vi "PeakFinder.vi"(9 "Trigger location":i32, 11 "Input Y values":dbl[](array[numeric])) -> (2 "peak?":bool, 3 "Input Y values":dbl[](array[numeric]))   [LabVIEW 2014]
panel:
  # "Peak Finder VI"
  # "Inputs"
  # "Outputs"
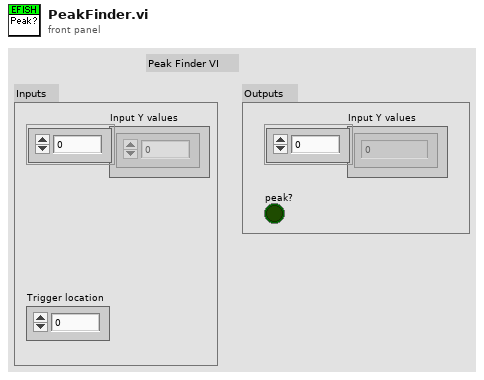
[diagram p1: front panel]
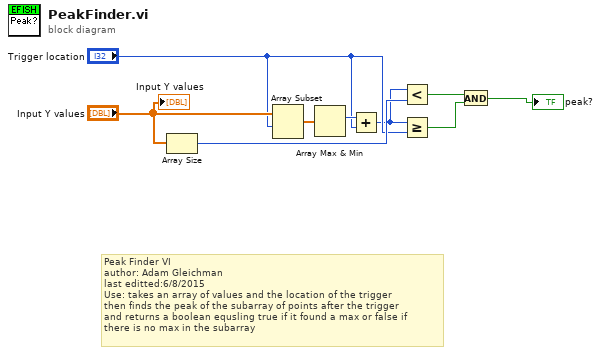
[diagram p0: block diagram]
diagram:
  # "Peak Finder VI\nauthor: Adam Gleichman\nlast editted:6/8/2015\nUse: takes an array of values and the location of the trigger\nthen finds the peak of the subarray of points after the trigger\nand returns a boolean equsling true if it found a max or false if \nthere is no max in the subarray"
  n1 = Array Size(array="Input Y values") -> (size(s)=w4:i32)
  n2 = Array Subset(array="Input Y values", index="Trigger location") -> (w9:dbl[])  [unwired: 1 in]
  n3 = Array Max & Min(array=w9) -> (max index (indices)=w8:i32)  [unwired: 3 out]
  n4 = Add(x=w8, y="Trigger location") -> (x+y=w2:i32)
  n5 = Less?(x=w2, y=w4) -> (x < y?=w7:bool)
  n6 = Greater Or Equal?(x=w2, y="Trigger location") -> (x >= y?=w6:bool)
  n7 = And(x=w7, y=w6) -> (x .and. y?=→"peak?":bool)
  "Input Y values" <- "Input Y values"
